vi "WriteData.vi"(0 "data":string[][](table), 1 "path":path) -> ()   [LabVIEW 2014]
panel:
  out "Array":string[](array[string])
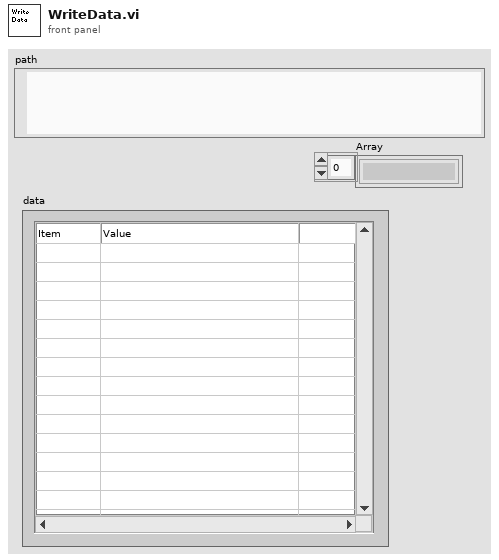
[diagram p1: front panel]
types:
  T1 = enum16{"open", "replace", "create", "open or create", "replace or create", "replace or create with confirmation"}
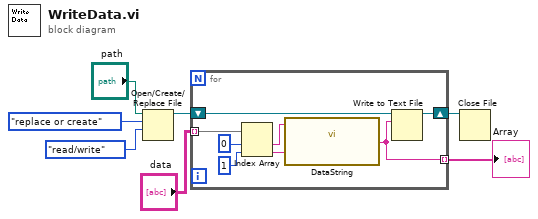
[diagram p0: block diagram]
diagram:
  n1 = Open/Create/Replace File(file path (use dialog)="path", operation (0:open)=T1."replace or create", access (0:read/write)=enum16{"read/write", "read-only", "write-only"}."read/write") -> (refnum out=w7:refnum<file>)  [unwired: 3 in, 2 out]
  n2 = for {
    shift-right: [w9] -> w5
    shift-left: w7 -> [w15]
    tunnel: "data" -> [w14] mode=indexing
    tunnel: [w8] -> w1 mode=indexing
    n3 = Index Array(array=w14, index #1=0 ("index"), index #2=1 ("index")) -> (element #1=w11:string, element #2=w10:string)
    n4 = call "DataString.vi"("Value"=w10, "Item"=w11) -> ("String"=w8:string)
    n5 = Write to Text File(file (use dialog)=w15, text=w8) -> (refnum out=w9:refnum<file>)  [unwired: 2 in, 2 out]
  }
  "Array" <- w1
  n6 = Close File(refnum=w5) -> ()  [unwired: 1 in, 2 out]
